vi "ip address.vi"() -> (3 "ip address":string)   [LabVIEW 2014]
uses:
  <vilib>/regexp/Match Regular Expression.xnode
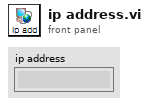
[diagram p1: front panel]
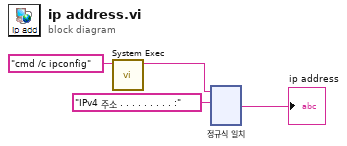
[diagram p0: block diagram]
diagram:
  n1 = call <vilib>:"System Exec.vi"("command line"="cmd /c ipconfig") -> ("standard output"=w2:string)  [unwired: 7 in, 3 out]
  n2 = xnode "정규식 일치"("입력 문자열"=w2, "정규식"="IPv4 주소 . . . . . . . . . :") -> ("일치 구문 뒤"=→"ip address":string)  [unwired: 4 in, 4 out]
